vi "Measurements Graph.vi"(0 "Bias Voltage":dbl[](array[numeric]), 2 "Stop_V":dbl, 5 "Resitance":dbl[](array[numeric]), 7 "Port 1 Cap":dbl[](array[numeric]), 9 "Port 2 Cap":dbl[](array[numeric]), 11 "Error In":errorcluster) -> (4 "Graph Cluster":T1, 15 "Error Out":errorcluster)   [LabVIEW 2013]
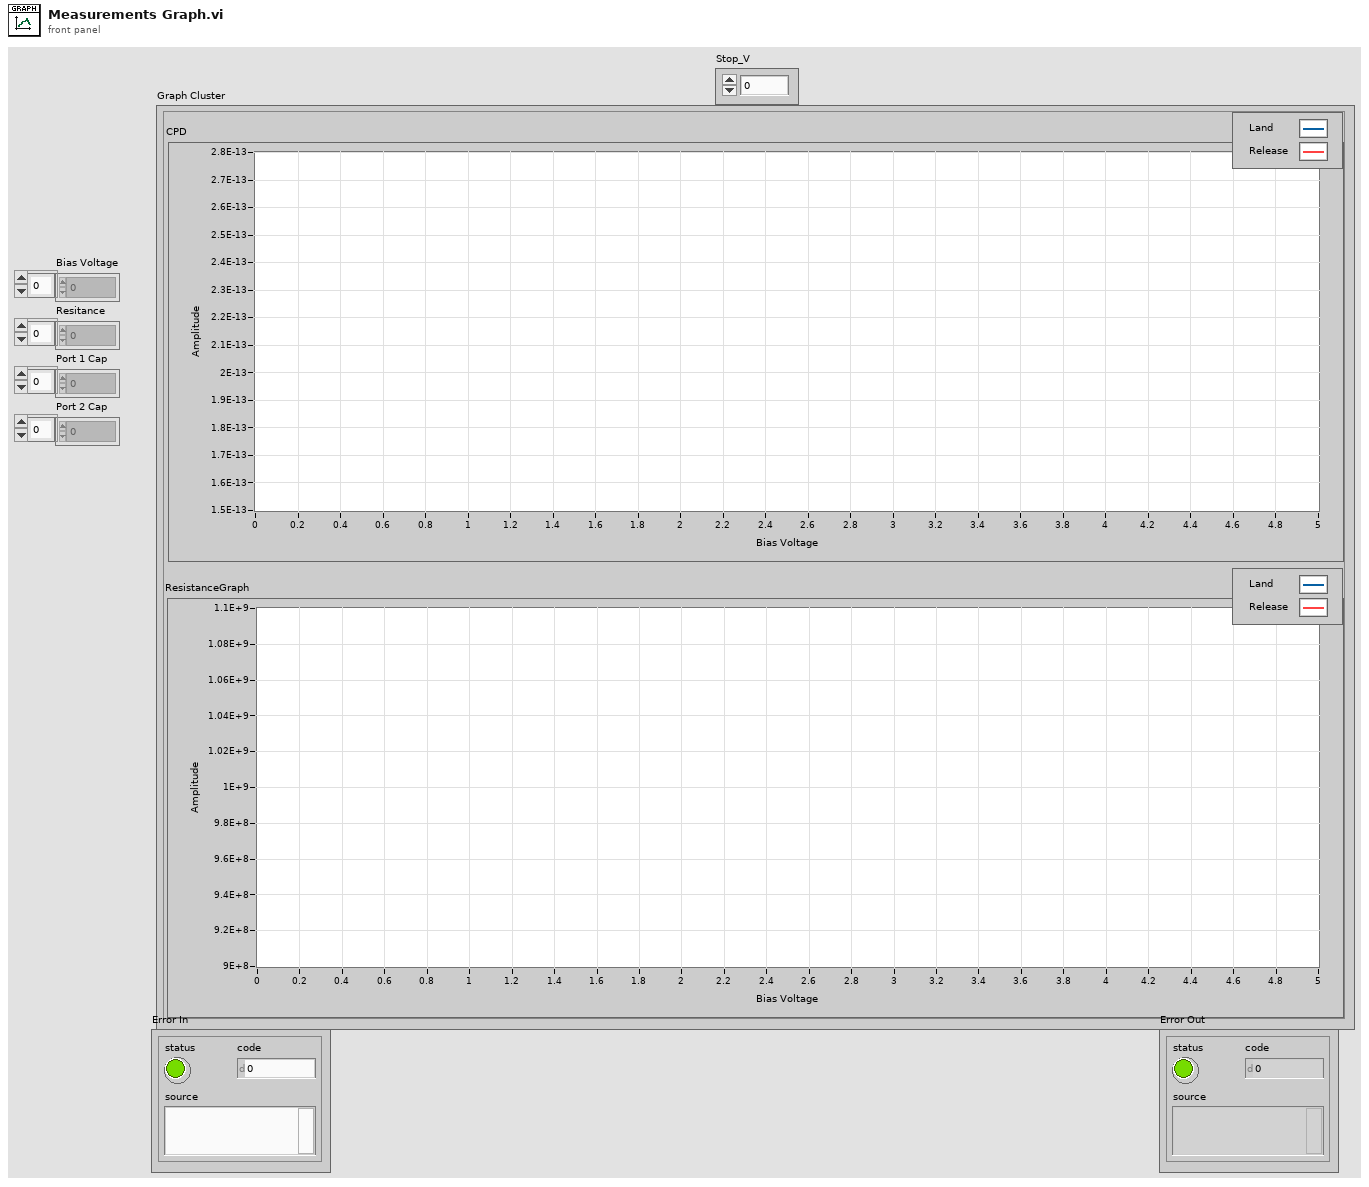
[diagram p1: front panel]
types:
  T1 = cluster{"ResistanceGraph":cluster{dbl[], dbl[]}[], "CPD":cluster{dbl[], dbl[]}[]}
  T2 = cluster{cluster{dbl[], dbl[]}[], cluster{dbl[], dbl[]}[]}
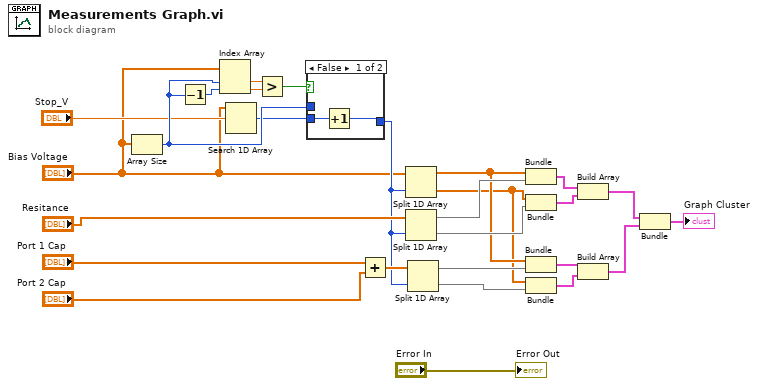
[diagram p0: block diagram]
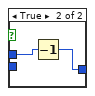
[diagram p2: hidden frame]
diagram:
  n1 = Array Size(array="Bias Voltage") -> (size(s)=w6:i32)
  n2 = Decrement(x=w6) -> (x-1=w9:i32)
  n3 = Index Array(array="Bias Voltage", index #1=w6, index #2=w9) -> (element #1=w7:dbl, element #2=w8:dbl)
  n4 = Search 1D Array(1D array="Bias Voltage", element="Stop_V") -> (index of element=w2:i32)  [unwired: 1 in]
  n5 = Greater?(x=w7, y=w8) -> (0:w1:bool)
  n6 = case shown="False" w1 {
    tunnel: w6 -> [_ w31]
    tunnel: [w28 w30] -> w5
    tunnel: w2 -> [w29 _]
    frame False {
      n7 = Increment(x=w29) -> (x+1=w28:i32)
    }
    frame True {
      n8 = Decrement(x=w31) -> (x-1=w30:i32)
    }
  }
  n9 = Add(x="Port 1 Cap", y="Port 2 Cap") -> (x+y=w18:dbl[])
  n10 = Split 1D Array(array="Bias Voltage", index=w5) -> (first subarray=w15:dbl[], second subarray=w14:dbl[])
  n11 = Split 1D Array(array="Resitance", index=w5) -> (first subarray=w26:dbl[], second subarray=w25:dbl[])
  n12 = Split 1D Array(array=w18, index=w5) -> (first subarray=w20:dbl[], second subarray=w19:dbl[])
  n13 = Bundle(w15, w26) -> (w24:cluster{dbl[], dbl[]})  [unwired: 1 in]
  n14 = Bundle(w14, w25) -> (w23:cluster{dbl[], dbl[]})  [unwired: 1 in]
  n15 = Bundle(w15, w20) -> (w22:cluster{dbl[], dbl[]})  [unwired: 1 in]
  n16 = Bundle(w14, w19) -> (w21:cluster{dbl[], dbl[]})  [unwired: 1 in]
  n17 = Build Array(w24, w23) -> (w13:cluster{dbl[], dbl[]}[])
  n18 = Build Array(w22, w21) -> (w12:cluster{dbl[], dbl[]}[])
  n19 = Bundle(w13, w12) -> (→"Graph Cluster":T2)  [unwired: 1 in]
  "Error Out" <- "Error In"
